vi "DBL to Bytes.vi"(11 "Numeric":dbl) -> (3 "ASIST DBL":string)   [LabVIEW 2018, in "TCPServer.lvlib"]
uses:
  TCPServer.lvlib
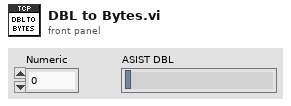
[diagram p1: front panel]
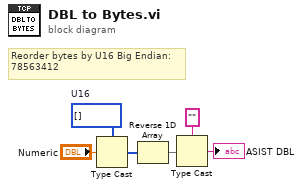
[diagram p0: block diagram]
diagram:
  w5 = u16[] []  # U16
  # "Reorder bytes by U16 Big Endian:\n78563412"
  n1 = Type Cast(type=w5, x="Numeric") -> (*(type *) &x=w6:u16[])
  n2 = Reverse 1D Array(array=w6) -> (reversed array=w3:u16[])
  n3 = Type Cast(type="", x=w3) -> (*(type *) &x=→"ASIST DBL":string)
